vi "G-Audio - Write Audio File.vi"() -> ()   [LabVIEW 2020]
uses:
  G-Audio/Controls/Audio File Info.ctl
  G-Audio/Controls/WAV Codec Specific Info.ctl
  G-Audio/Controls/WAV Container Format.ctl
  G-Audio/Controls/WAV Data Format.ctl
  904fc059-1fb5-4948-99d7-f152d287243f.vi
  G-Audio/Polymorphic VIs/Open Audio File Write (WAV).vi
  47f0ab39-b770-4e11-8653-c44c5d8a6007.vi
  cc8aa77b-4c14-46cf-bd44-a282a9601a61.vi
  32d52177-6bf5-4367-8f35-be0c7c0cfd33.vi
  <vilib>/Analysis/1siggen.llb/Ramp Pattern.vi
  <vilib>/Analysis/1siggen.llb/Ramp Pattern by Samples.vi
  904fc059-1fb5-4948-99d7-f152d287243f.vi/893057dd-ddaa-4be7-9dc5-db20c1d3eef0.vi
  G-Audio/Private/Get Codec.vi
  G-Audio/Private/Result To Error.vi
  47f0ab39-b770-4e11-8653-c44c5d8a6007.vi/fba40667-3e21-44fa-934c-95909d78721c.vi
  cc8aa77b-4c14-46cf-bd44-a282a9601a61.vi/fba40667-3e21-44fa-934c-95909d78721c.vi
  32d52177-6bf5-4367-8f35-be0c7c0cfd33.vi/fba40667-3e21-44fa-934c-95909d78721c.vi
  G-Audio/Private/Get File Extension (Reentrant).vi
  47f0ab39-b770-4e11-8653-c44c5d8a6007.vi/fba40667-3e21-44fa-934c-95909d78721c.vi/4b7b629c-2e91-4160-9820-a26af8f6e677.vi
  47f0ab39-b770-4e11-8653-c44c5d8a6007.vi/fba40667-3e21-44fa-934c-95909d78721c.vi/e7c4a249-ce38-42b4-8985-5fdb76b4ebfc.vi
  cc8aa77b-4c14-46cf-bd44-a282a9601a61.vi/fba40667-3e21-44fa-934c-95909d78721c.vi/4b7b629c-2e91-4160-9820-a26af8f6e677.vi
  cc8aa77b-4c14-46cf-bd44-a282a9601a61.vi/fba40667-3e21-44fa-934c-95909d78721c.vi/e7c4a249-ce38-42b4-8985-5fdb76b4ebfc.vi
  32d52177-6bf5-4367-8f35-be0c7c0cfd33.vi/fba40667-3e21-44fa-934c-95909d78721c.vi/4b7b629c-2e91-4160-9820-a26af8f6e677.vi
  32d52177-6bf5-4367-8f35-be0c7c0cfd33.vi/fba40667-3e21-44fa-934c-95909d78721c.vi/e7c4a249-ce38-42b4-8985-5fdb76b4ebfc.vi
  <vilib>/measure/masignal.llb/Sine Waveform.vi
  <vilib>/Utility/error.llb/Error Cluster From Error Code.vi
  G-Audio/G-Audio.lvlib
panel:
  out "error out":errorcluster
  # "Instructions:\n1. Run the VI.\n2. Select a location to save the WAV file.\n3. A short WAV file will be saved containing a 220Hz sine function.\n4. Listen to the WAV with the G-Audio - Continuous Output.vi example."
  # "G"
  # "-Audio"
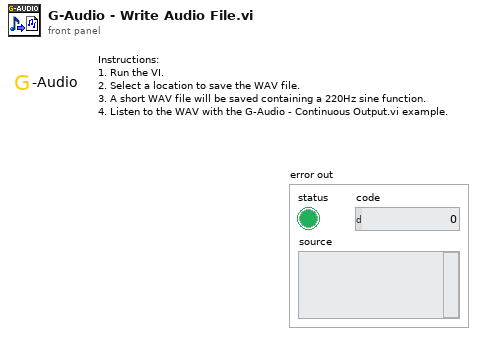
[diagram p1: front panel]
types:
  T1 = typedef "G-Audio.lvlib/WAV Codec Specific Info.ctl" = cluster{"Container Format":T2, "Data Format":T3}
  T2 = typedef "G-Audio.lvlib/WAV Container Format.ctl" = enum32{"RIFF", "Wave64"}
  T3 = typedef "G-Audio.lvlib/WAV Data Format.ctl" = u32
  T4 = typedef "G-Audio.lvlib/Audio File Info.ctl" = cluster{"Sample Rate (Hz)":u32, "Channels":u32, "Bit Depth":u32}
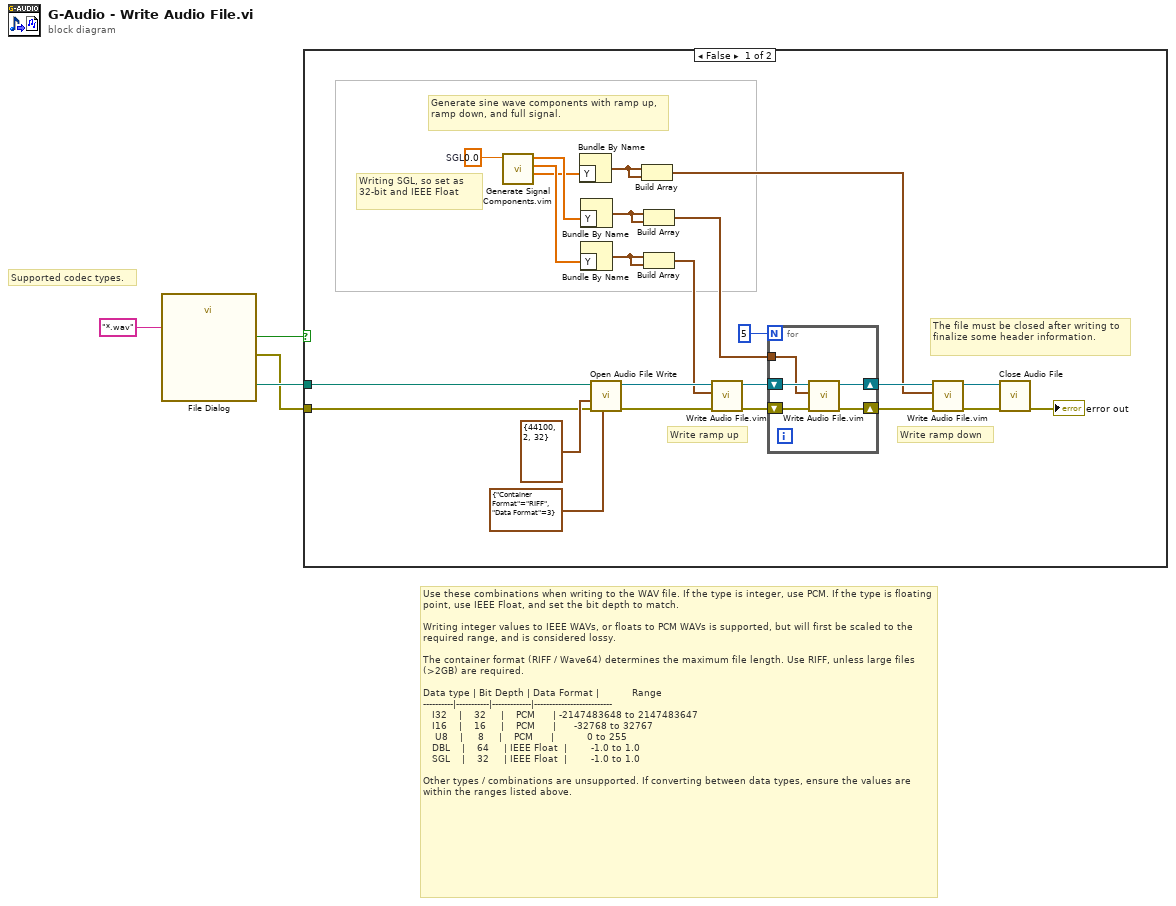
[diagram p0: block diagram]
diagram:
  # "Supported codec types."
  # "Use these combinations when writing to the WAV file. If the type is integer, use PCM. If the type is floating point, use IEEE Float, and set the bit depth to match.\n\nWriting integer values to IEEE WAVs, or floats to PCM WAVs is supported, but will first be scaled to the required range, and is considered lossy.\n\nThe container format (RIFF / Wave64) determines the maximum file length. Use RIFF, unless large files (>2GB) are required.\n\nData type | Bit Depth | Data Format |           Range\n----------|-----------|-------------|--------------------------\n   I32    |    32     |    PCM      | -2147483648 to 2147483647\n   I16    |    16     |    PCM      |      -32768 to 32767\n    U8    |     8     |    PCM      |           0 to 255\n   DBL    |    64     | IEEE Float  |        -1.0 to 1.0\n   SGL    |    32     | IEEE Float  |        -1.0 to 1.0\n\nOther types / combinations are unsupported. If converting between data types, ensure the values are within the ranges listed above."
  n1 = call "File Dialog"("pattern (all files)"="*.wav") -> ("selected path"=w3:path, "cancelled"=w1:bool, "error out"=w2:errorcluster)  [unwired: 11 in, 1 out]
  n2 = case shown="False" w1 {
    tunnel: w3 -> [w26 _]
    tunnel: w2 -> [w24 _]
    frame False {
      w5 = sgl 0.0  # SGL
      # "Generate sine wave components with ramp up, ramp down, and full signal."
      # "Writing SGL, so set as 32-bit and IEEE Float"
      # "Write ramp down"
      # "Write ramp up"
      # "The file must be closed after writing to finalize some header information."
      n3 = call "Generate Signal Components.vim"("Data Type"=w5) -> ("Ramp Down"=w9:sgl[], "Ramp Up"=w13:sgl[], "Signal"=w11:sgl[])  [unwired: 8 in]
      n4 = Bundle By Name("Y"=w9) -> (w8:waveform(sgl))  [unwired: 1 in]
      n5 = Bundle By Name("Y"=w11) -> (w10:waveform(sgl))  [unwired: 1 in]
      n6 = Bundle By Name("Y"=w13) -> (w12:waveform(sgl))  [unwired: 1 in]
      n7 = call-poly "Open Audio File Write.vi"("Codec Specific Info"=T1 {"Container Format"=enum."RIFF", "Data Format"=3} ("WAV File Info"), "error in (no error)"=w24, "Audio File Info"=T4 {"Sample Rate (Hz)"=44100, "Channels"=2, "Bit Depth"=32}, "Path"=w26) -> ("error out"=w21:errorcluster, "Audio File Refnum"=w23:refnum<file>)  [unwired: 6 in]
      n8 = Build Array(w8, w8) -> (w14:waveform(sgl)[])
      n9 = Build Array(w10, w10) -> (w6:waveform(sgl)[])
      n10 = Build Array(w12, w12) -> (w7:waveform(sgl)[])
      n11 = call "Write Audio File.vim"("error in (no error)"=w21, "Audio Data"=w7, "Audio File Refnum In"=w23) -> ("error out"=w20:errorcluster, "Audio File Refnum Out"=w22:refnum<file>)  [unwired: 7 in]
      n12 = for {
        N: 5 -> [_]
        shift-right: [w33] -> w16
        shift-left: w22 -> [w31]
        shift-right: [w32] -> w18
        shift-left: w20 -> [w30]
        tunnel: w6 -> [w29]
        n13 = call "Write Audio File.vim"("error in (no error)"=w30, "Audio Data"=w29, "Audio File Refnum In"=w31) -> ("error out"=w32:errorcluster, "Audio File Refnum Out"=w33:refnum<file>)  [unwired: 7 in]
      }
      n14 = call "Write Audio File.vim"("error in (no error)"=w18, "Audio Data"=w14, "Audio File Refnum In"=w16) -> ("error out"=w17:errorcluster, "Audio File Refnum Out"=w15:refnum<file>)  [unwired: 7 in]
      n15 = call "Close Audio File.vi"("error in (no error)"=w17, "Audio File Refnum In"=w15) -> ("error out"=→"error out":errorcluster)  [unwired: 9 in]
    }
    frame True {
    }
  }
